vi "3.1.1-VectorNav.vi"() -> ()   [LabVIEW 2010]
panel:
  in  "stop":bool
  out "Serial Settings:Number of Bytes at Serial Port":u32
  out "read buffer":string
  out "return count":u32
  in  "VISA resource name":refnum<visa-resource-name>
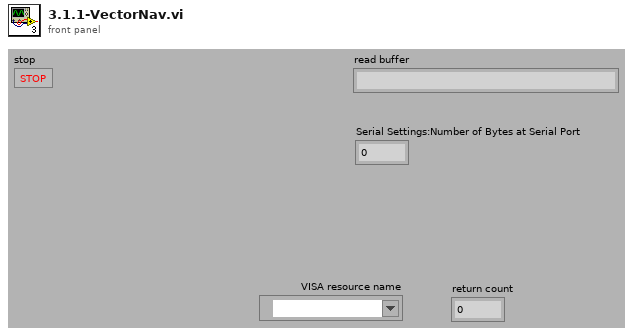
[diagram p1: front panel]
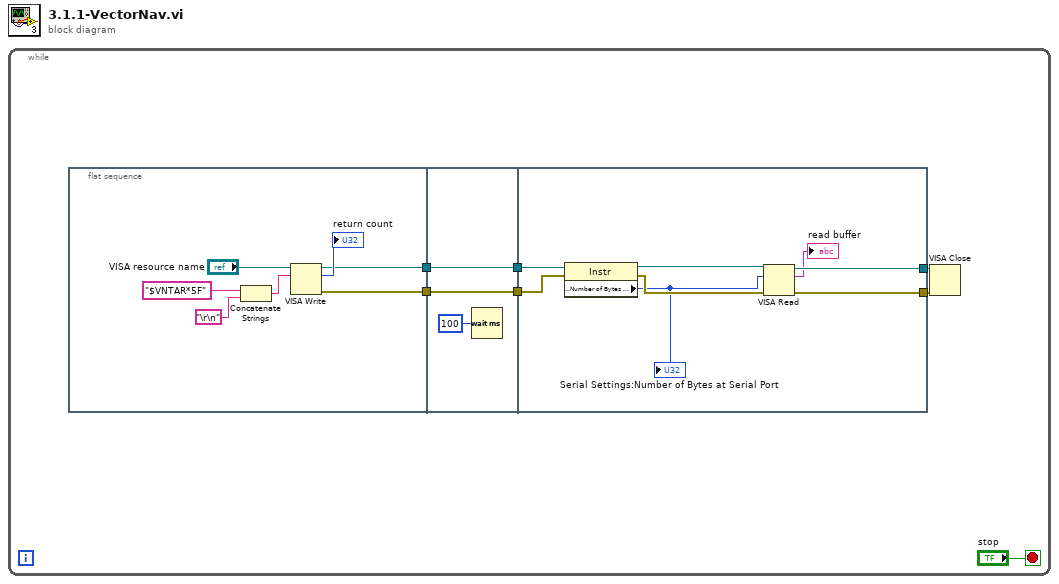
[diagram p0: block diagram]
diagram:
  n1 = while {
    stop <- "stop" stop-if-true
    n2 = flat-sequence {
      tunnel: [w9] -> w4
      tunnel: [w8] -> w2
      tunnel: w4 -> [w17]
      tunnel: [w17] -> w3
      tunnel: w2 -> [w16]
      tunnel: [w16] -> w1
      tunnel: w3 -> [w22]
      tunnel: w1 -> [w21]
      tunnel: [w25] -> w7
      tunnel: [w24] -> w6
      frame #0 {
        n3 = Concatenate Strings("$VNTAR*5F" ("write buffer"), "\r\n") -> (w10:string)
        n4 = VISA Write(VISA resource name="VISA resource name", write buffer=w10) -> (VISA resource name out=w9:refnum<visa-resource-name>, return count=→"return count":u32, error out=w8:errorcluster)  [unwired: 1 in]
      }
      frame #1 {
        n5 = Wait (ms)(milliseconds to wait=u32 100) -> ()  [unwired: 1 out]
      }
      frame #2 {
        n6 = property class="Instr"(reference=w22, error in=w21) -> (reference out=w20:refnum<visa-resource-name>, error out=w19:errorcluster, "Serial Settings:Number of Bytes at Serial Port"=w18:u32)
        "Serial Settings:Number of Bytes at Serial Port" <- w18
        n7 = VISA Read(VISA resource name=w20, byte count=w18, error in (no error)=w19) -> (VISA resource name out=w25:refnum<visa-resource-name>, read buffer=→"read buffer":string, error out=w24:errorcluster)  [unwired: 1 out]
      }
    }
    n8 = VISA Close(VISA resource name=w7, error in (no error)=w6) -> ()  [unwired: 1 out]
  }
